vi "Return_Data.vi"(8 "error in (no error)":errorcluster caption="entrée d'erreur (pas d'erreur)", 11 "Class Relay_Board en entrée":refnum<class "Class Instrument UART.lvclass">) -> (0 "error out":errorcluster caption="sortie d'erreur", 2 "Data_Json":string, 3 "Class Relay_Board en Sortie":refnum<class "Class Instrument UART.lvclass">)   [LabVIEW 2020, in "Library Instrument & Equipement.lvlib" / "Library Instruments.lvlib" / "Class Instrument UART.lvclass"]
uses:
  Class Instrument UART.lvclass
  Class Instrument UART.lvclass/Class Instrument UART.ctl
  JSON API/Variant JSON/Variant to JSON.vi
  JSON API/JSON Value/Get Item by name array.vi
  UART/UART (Default)/Class UART (Default).lvclass
  JSON API/JSON Value/JSON Value.lvclass
  JSON API/Get Polymorphic/JSON GetSet.lvlib
  JSON API/Variant JSON/Variant JSON.lvlib
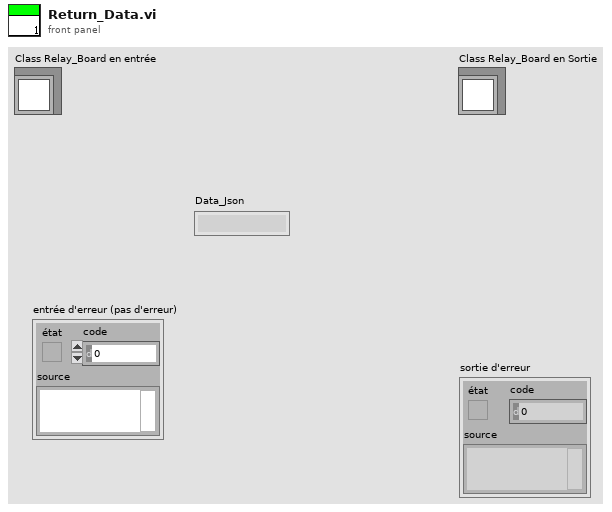
[diagram p1: front panel]
types:
  T1 = cluster{"Frame Read":string, "Frame received":bool, "Frame NOk":bool}
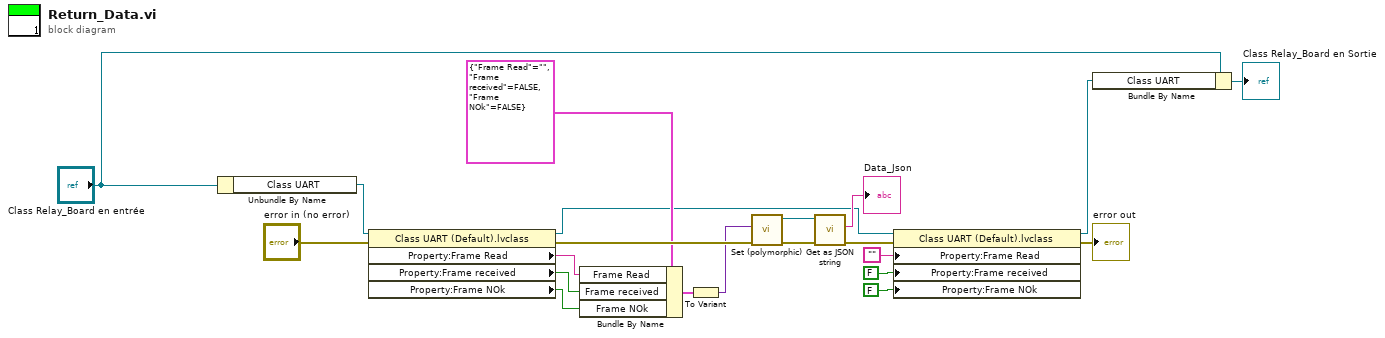
[diagram p0: block diagram]
diagram:
  n1 = Unbundle By Name("Class Relay_Board en entrée") -> ("Class UART"=w20:refnum<class "Class UART (Default).lvclass">)
  n2 = property class="Class UART (Default).lvclass"(reference=w20, error in="error in (no error)") -> (reference out=w7:refnum<class "Class UART (Default).lvclass">, error out=w18:errorcluster, "Property:Frame Read"=w13:string, "Property:Frame received"=w12:bool, "Property:Frame NOk"=w11:bool)
  n3 = Bundle By Name(cluster=T1 {"Frame Read"="", "Frame received"=FALSE, "Frame NOk"=FALSE}, "Frame Read"=w13, "Frame received"=w12, "Frame NOk"=w11) -> (w10:T1)
  n4 = To Variant(anything=w10) -> (Variant=w15:variant)
  n5 = call-poly "Set (polymorphic).vi"("error in (no error)"=w18, "Variant"=w15) -> ("error out"=w16:errorcluster, "JSON Value out"=w17:refnum<class "JSON Value.lvclass">)  [unwired: 8 in]
  n6 = call "Get as JSON string.vi"("error in (no error)"=w16, "JSON Value in"=w17) -> ("error out"=w9:errorcluster, "<JSON>"=→"Data_Json":string)  [unwired: 8 in]
  n7 = property class="Class UART (Default).lvclass"(reference=w7, error in=w9, "Property:Frame Read"="", "Property:Frame received"=FALSE ("Frame received"), "Property:Frame NOk"=FALSE ("Frame NOk")) -> (reference out=w5:refnum<class "Class UART (Default).lvclass">, error out=→"error out":errorcluster)
  n8 = Bundle By Name(cluster="Class Relay_Board en entrée", "Class UART"=w5) -> (→"Class Relay_Board en Sortie":refnum<class "Class Instrument UART.lvclass">)
